vi "HOST.vi"() -> ()   [LabVIEW 2018]
uses:
  <vilib>/userdefined/High Color/nirio_resource_hc.ctl
  <vilib>/FPGAPlugInAG/PXI-7953R/niLvFpga_Open_PXI-7953R.vi
  <vilib>/rvi/interface/common/dynamic/niFpgaDynamicAddResources.vi
  <vilib>/FPGAPlugInAG/Dynamic/niLvFpga_Reset_Dynamic.vi
  <vilib>/FPGAPlugInAG/Dynamic/niLvFpga_Run_Dynamic.vi
  <vilib>/Utility/error.llb/Error Cluster From Error Code.vi
  <vilib>/rvi/errors/niLvFpgaAdjustHostInterfaceError.vi
  <vilib>/rvi/interface/nirviOpenFPGA/nirviOpenFPGA.xnode
  FPGA Bitfiles/Testfor6581_FPGATarget_Testfor6581_i4r3kXWw-5U.lvbitx
  <vilib>/rvi/interface/nirviMethod/nirviMethod.xnode
  <vilib>/rvi/interface/nirviReadWriteControl/nirviReadWriteControl.xnode
  NiFpgaLv.dll
  <vilib>/rvi/interface/Simulation/niFpgaSimulationCallBeginRW.vi
panel:
  in  "IO Module\\DDCB_PFI3_Write":bool
  in  "IO Module\\DDCB_PFI2_Write":bool
  in  "IO Module\\DDCB_PFI1_Write":bool
  in  "IO Module\\DDCB_DIO23_Write":bool
  in  "IO Module\\DDCB_DIO22_Write":bool
  in  "IO Module\\DDCB_DIO21_Write":bool
  in  "IO Module\\DDCB_DIO20_Write":bool
  in  "IO Module\\DDCB_DIO19_Write":bool
  in  "IO Module\\DDCB_DIO18_Write":bool
  in  "IO Module\\DDCB_DIO17_Write":bool
  in  "IO Module\\DDCB_DIO16_Write":bool
  in  "IO Module\\DDCB_DIO15_Write":bool
  in  "IO Module\\DDCB_DIO14_Write":bool
  in  "IO Module\\DDCB_DIO13_Write":bool
  in  "IO Module\\DDCB_DIO12_Write":bool
  in  "IO Module\\DDCB_DIO11_Write":bool
  in  "IO Module\\DDCB_DIO10_Write":bool
  in  "IO Module\\DDCB_DIO9_Write":bool
  in  "IO Module\\DDCB_DIO8_Write":bool
  in  "IO Module\\DDCB_DIO7_Write":bool
  in  "IO Module\\DDCB_DIO6_Write":bool
  in  "IO Module\\DDCB_DIO5_Write":bool
  in  "IO Module\\DDCB_DIO4_Write":bool
  in  "IO Module\\DDCB_DIO3_Write":bool
  in  "IO Module\\DDCB_DIO2_Write":bool
  in  "IO Module\\DDCB_DIO1_Write":bool
  in  "IO Module\\DDCB_DIO0_Write":bool
  in  "IO Module\\DDCA_PFI3_Write":bool
  in  "IO Module\\DDCA_PFI2_Write":bool
  in  "IO Module\\DDCA_PFI1_Write":bool
  in  "IO Module\\DDCA_DIO23_Write":bool
  in  "IO Module\\DDCA_DIO22_Write":bool
  in  "IO Module\\DDCA_DIO21_Write":bool
  in  "IO Module\\DDCA_DIO20_Write":bool
  in  "IO Module\\DDCA_DIO19_Write":bool
  in  "IO Module\\DDCA_DIO18_Write":bool
  in  "IO Module\\DDCA_DIO17_Write":bool
  in  "IO Module\\DDCA_DIO16_Write":bool
  in  "IO Module\\DDCA_DIO15_Write":bool
  in  "IO Module\\DDCA_DIO14_Write":bool
  in  "IO Module\\DDCA_DIO13_Write":bool
  in  "IO Module\\DDCA_DIO12_Write":bool
  in  "IO Module\\DDCA_DIO11_Write":bool
  in  "IO Module\\DDCA_DIO10_Write":bool
  in  "IO Module\\DDCA_DIO9_Write":bool
  in  "IO Module\\DDCA_DIO8_Write":bool
  in  "IO Module\\DDCA_DIO7_Write":bool
  in  "IO Module\\DDCA_DIO6_Write":bool
  in  "IO Module\\DDCA_DIO5_Write":bool
  in  "IO Module\\DDCA_DIO4_Write":bool
  in  "IO Module\\DDCA_DIO3_Write":bool
  in  "IO Module\\DDCA_DIO2_Write":bool
  in  "IO Module\\DDCA_DIO1_Write":bool
  in  "IO Module\\DDCA_DIO0_Write":bool
  in  "Стоп":bool
  in  "resource name":T1="PXI1Slot6"
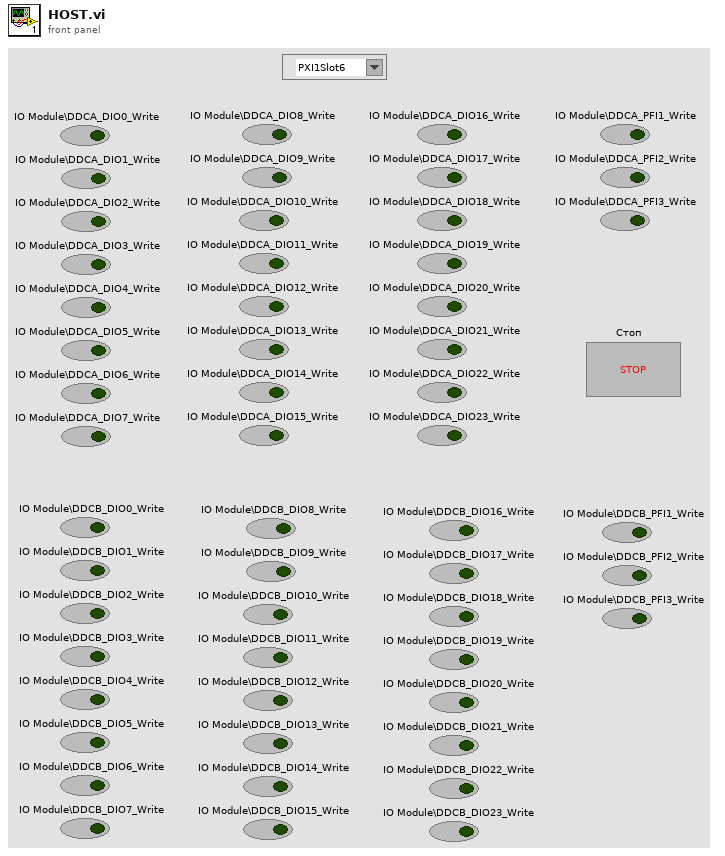
[diagram p1: front panel]
types:
  T1 = typedef "nirio_resource_hc.ctl" = tag
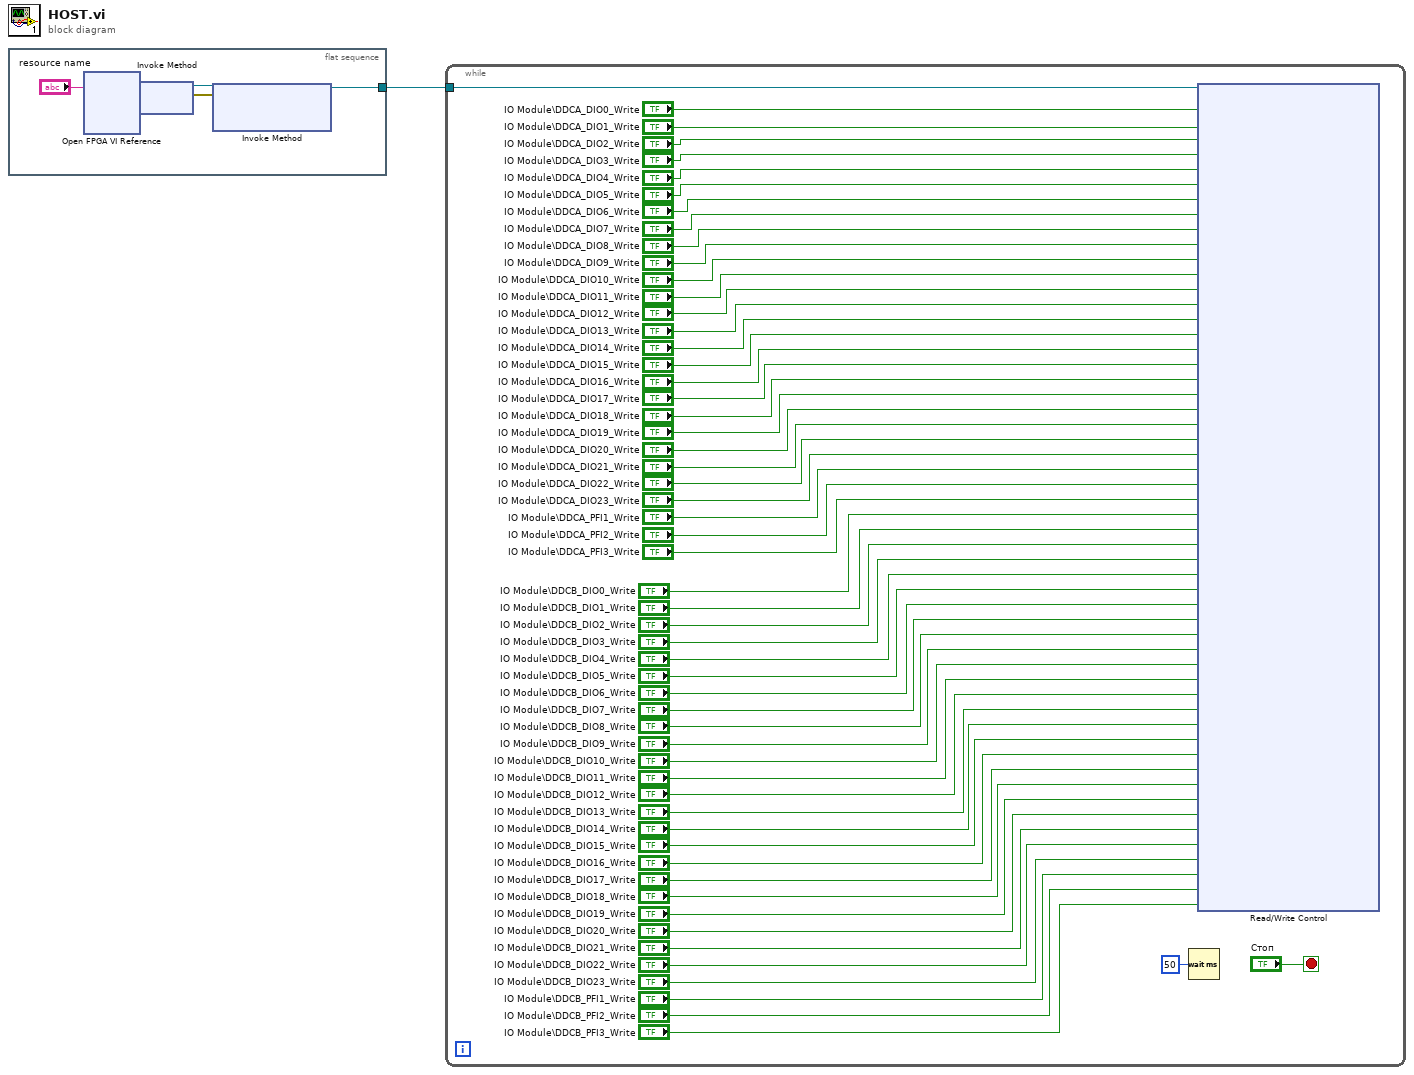
[diagram p0: block diagram]
diagram:
  n1 = flat-sequence {
    tunnel: [w2] -> w1
    frame #0 {
      n2 = xnode "Open FPGA VI Reference"("resource name"="resource name") -> ("FPGA VI Reference Out"=w3:refnum<k20>, "error out"=w5:errorcluster)  [unwired: 1 in]
      n3 = xnode "Invoke Method"("FPGA VI Reference In"=w3, "error in"=w5) -> ("FPGA VI Reference Out"=w6:refnum<k20>, "error out"=w4:errorcluster)
      n4 = xnode "Invoke Method"("FPGA VI Reference In"=w6, "error in"=w4) -> ("FPGA VI Reference Out"=w2:refnum<k20>)  [unwired: 1 in, 1 out]
    }
  }
  n5 = while {
    tunnel: w1 -> [w62]
    stop <- "Стоп" stop-if-true
    n6 = Wait (ms)(milliseconds to wait=u32 50) -> ()  [unwired: 1 out]
    n7 = xnode "Read/Write Control"("FPGA VI Reference In"=w62, "IO Module\\DDCA_DIO0_Write"="IO Module\\DDCA_DIO0_Write", "IO Module\\DDCA_DIO1_Write"="IO Module\\DDCA_DIO1_Write", "IO Module\\DDCA_DIO2_Write"="IO Module\\DDCA_DIO2_Write", "IO Module\\DDCA_DIO3_Write"="IO Module\\DDCA_DIO3_Write", "IO Module\\DDCA_DIO4_Write"="IO Module\\DDCA_DIO4_Write", "IO Module\\DDCA_DIO5_Write"="IO Module\\DDCA_DIO5_Write", "IO Module\\DDCA_DIO6_Write"="IO Module\\DDCA_DIO6_Write", "IO Module\\DDCA_DIO7_Write"="IO Module\\DDCA_DIO7_Write", "IO Module\\DDCA_DIO8_Write"="IO Module\\DDCA_DIO8_Write", "IO Module\\DDCA_DIO9_Write"="IO Module\\DDCA_DIO9_Write", "IO Module\\DDCA_DIO10_Write"="IO Module\\DDCA_DIO10_Write", "IO Module\\DDCA_DIO11_Write"="IO Module\\DDCA_DIO11_Write", "IO Module\\DDCA_DIO12_Write"="IO Module\\DDCA_DIO12_Write", "IO Module\\DDCA_DIO13_Write"="IO Module\\DDCA_DIO13_Write", "IO Module\\DDCA_DIO14_Write"="IO Module\\DDCA_DIO14_Write", "IO Module\\DDCA_DIO15_Write"="IO Module\\DDCA_DIO15_Write", "IO Module\\DDCA_DIO16_Write"="IO Module\\DDCA_DIO16_Write", "IO Module\\DDCA_DIO17_Write"="IO Module\\DDCA_DIO17_Write", "IO Module\\DDCA_DIO18_Write"="IO Module\\DDCA_DIO18_Write", "IO Module\\DDCA_DIO19_Write"="IO Module\\DDCA_DIO19_Write", "IO Module\\DDCA_DIO20_Write"="IO Module\\DDCA_DIO20_Write", "IO Module\\DDCA_DIO21_Write"="IO Module\\DDCA_DIO21_Write", "IO Module\\DDCA_DIO22_Write"="IO Module\\DDCA_DIO22_Write", "IO Module\\DDCA_DIO23_Write"="IO Module\\DDCA_DIO23_Write", "IO Module\\DDCA_PFI1_Write"="IO Module\\DDCA_PFI1_Write", "IO Module\\DDCA_PFI2_Write"="IO Module\\DDCA_PFI2_Write", "IO Module\\DDCA_PFI3_Write"="IO Module\\DDCA_PFI3_Write", "IO Module\\DDCB_DIO0_Write"="IO Module\\DDCB_DIO0_Write", "IO Module\\DDCB_DIO1_Write"="IO Module\\DDCB_DIO1_Write", "IO Module\\DDCB_DIO2_Write"="IO Module\\DDCB_DIO2_Write", "IO Module\\DDCB_DIO3_Write"="IO Module\\DDCB_DIO3_Write", "IO Module\\DDCB_DIO4_Write"="IO Module\\DDCB_DIO4_Write", "IO Module\\DDCB_DIO5_Write"="IO Module\\DDCB_DIO5_Write", "IO Module\\DDCB_DIO6_Write"="IO Module\\DDCB_DIO6_Write", "IO Module\\DDCB_DIO7_Write"="IO Module\\DDCB_DIO7_Write", "IO Module\\DDCB_DIO8_Write"="IO Module\\DDCB_DIO8_Write", "IO Module\\DDCB_DIO9_Write"="IO Module\\DDCB_DIO9_Write", "IO Module\\DDCB_DIO10_Write"="IO Module\\DDCB_DIO10_Write", "IO Module\\DDCB_DIO11_Write"="IO Module\\DDCB_DIO11_Write", "IO Module\\DDCB_DIO12_Write"="IO Module\\DDCB_DIO12_Write", "IO Module\\DDCB_DIO13_Write"="IO Module\\DDCB_DIO13_Write", "IO Module\\DDCB_DIO14_Write"="IO Module\\DDCB_DIO14_Write", "IO Module\\DDCB_DIO15_Write"="IO Module\\DDCB_DIO15_Write", "IO Module\\DDCB_DIO16_Write"="IO Module\\DDCB_DIO16_Write", "IO Module\\DDCB_DIO17_Write"="IO Module\\DDCB_DIO17_Write", "IO Module\\DDCB_DIO18_Write"="IO Module\\DDCB_DIO18_Write", "IO Module\\DDCB_DIO19_Write"="IO Module\\DDCB_DIO19_Write", "IO Module\\DDCB_DIO20_Write"="IO Module\\DDCB_DIO20_Write", "IO Module\\DDCB_DIO21_Write"="IO Module\\DDCB_DIO21_Write", "IO Module\\DDCB_DIO22_Write"="IO Module\\DDCB_DIO22_Write", "IO Module\\DDCB_DIO23_Write"="IO Module\\DDCB_DIO23_Write", "IO Module\\DDCB_PFI1_Write"="IO Module\\DDCB_PFI1_Write", "IO Module\\DDCB_PFI2_Write"="IO Module\\DDCB_PFI2_Write", "IO Module\\DDCB_PFI3_Write"="IO Module\\DDCB_PFI3_Write") -> ()  [unwired: 1 in, 2 out]
  }
